vi "TEST_bench_mean_of_FIFO.vi"() -> ()   [LabVIEW 2017]
panel:
  out "FIFO_data":fxp<+/-,16,5>[](array[numeric])
  out "Array":fxp<+/-,33,22>[](array[numeric])
  in  "zk_s":fxp<+/-,33,22>[](array[numeric])
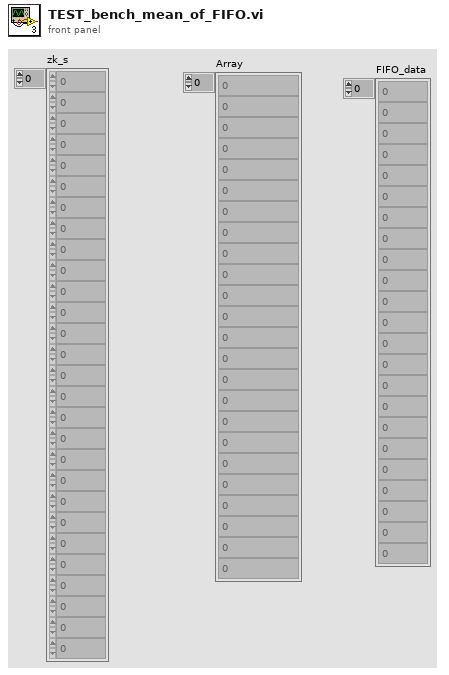
[diagram p1: front panel]
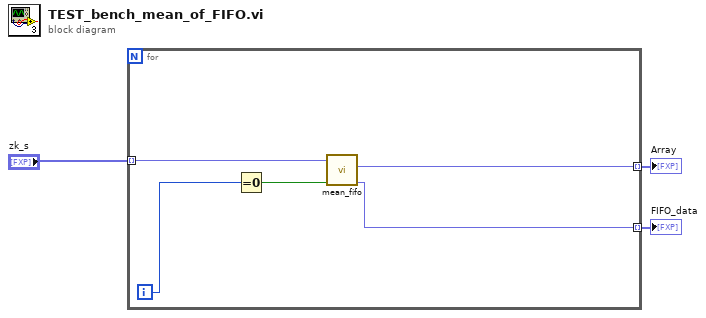
[diagram p0: block diagram]
diagram:
  n1 = for {
    tunnel: [w8] -> w2 mode=indexing
    tunnel: "zk_s" -> [w7] mode=indexing
    tunnel: [w6] -> w1 mode=indexing
    i -> [w4]
    n2 = Equal To 0?(x=w4) -> (x = 0?=w5:bool)
    n3 = call "mean_fifo.vi"("reset"=w5, "zk"=w7) -> ("fifo_data"=w6:fxp<+/-,16,5>, "mean"=w8:fxp<+/-,33,22>)  [unwired: 8 in]
  }
  "Array" <- w2
  "FIFO_data" <- w1
